vi "校准时拍照自动存图.vi"(11 "Img输入":T1) -> ()   [LabVIEW 2014]
uses:
  <vilib>/vision/Image Controls.llb/IMAQ Image.ctl
  Global.vi
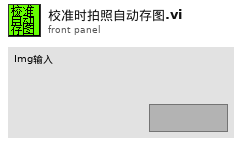
[diagram p1: front panel]
types:
  T1 = typedef "IMAQ Image.ctl" = refnum<image>
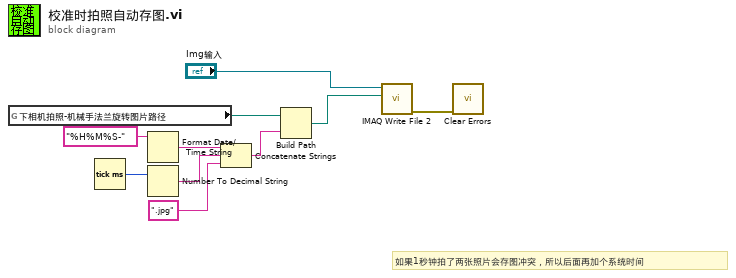
[diagram p0: block diagram]
diagram:
  # "如果1秒钟拍了两张照片会存图冲突，所以后面再加个系统时间"
  n1 = global read "Global.vi" "下相机拍照-机械手法兰旋转图片路径"() -> (w8:path)
  n2 = Tick Count (ms)() -> (millisecond timer value=w4:u32)
  n3 = Format Date/Time String(time format string (%c)="%H%M%S-") -> (date/time string=w6:string)  [unwired: 2 in]
  n4 = Number To Decimal String(number=w4) -> (decimal integer string=w3:string)  [unwired: 1 in]
  n5 = Concatenate Strings(w6, w3, ".jpg" ("字符串")) -> (w5:string)
  n6 = Build Path(base path=w8, name or relative path=w5) -> (appended path=w7:path)
  n7 = call-poly "IMAQ Write File 2"("File Path"=w7, "Image"="Img输入") -> ("error out"=w2:errorcluster)  [unwired: 8 in, 1 out]
  n8 = call <vilib>:"Clear Errors.vi"("error in (no error)"=w2) -> ()  [unwired: 5 in, 2 out]
